vi "OVERRISE-VAR.vi"() -> ()   [LabVIEW 2017]
panel:
  in  "Array 2":bool[](array[boolean])
  in  "Array":dbl[](array[numeric])
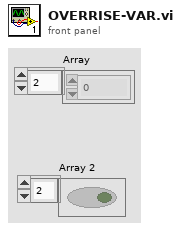
[diagram p1: front panel]
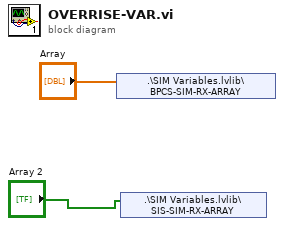
[diagram p0: block diagram]
diagram:
  n1 = shared-variable ".\\SIM Variables.lvlib\\BPCS-SIM-RX-ARRAY"("Array") -> ()  [unwired: 1 in, 1 out]
  n2 = shared-variable ".\\SIM Variables.lvlib\\SIS-SIM-RX-ARRAY"("Array 2") -> ()  [unwired: 1 in, 1 out]
